vi "Convert C to F.vi"(1 "摄氏温标":dbl) -> (0 "华氏温标":dbl)   [LabVIEW 2012]
doc: "该VI会将摄氏温度值转化为华氏温度值。"
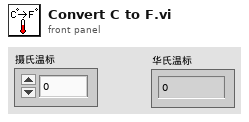
[diagram p1: front panel]
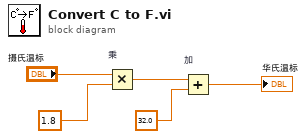
[diagram p0: block diagram]
diagram:
  n1 = Multiply "乘"(x="摄氏温标", y=1.8) -> (x*y=w3:dbl)
  n2 = Add "加"(x=w3, y=32.0) -> (x+y=→"华氏温标":dbl)
